vi "StageMoveDone.vi"(8 "error in (no error)":errorcluster, 11 "InterferometryUI in":refnum<class "InterferometryUI.lvclass">) -> (0 "error out":errorcluster, 3 "InterferometryUI out":refnum<class "InterferometryUI.lvclass">)   [LabVIEW 2023, in "InterferometryUI.lvlib" / "InterferometryUI.lvclass"]
uses:
  InterferometryUI.lvclass
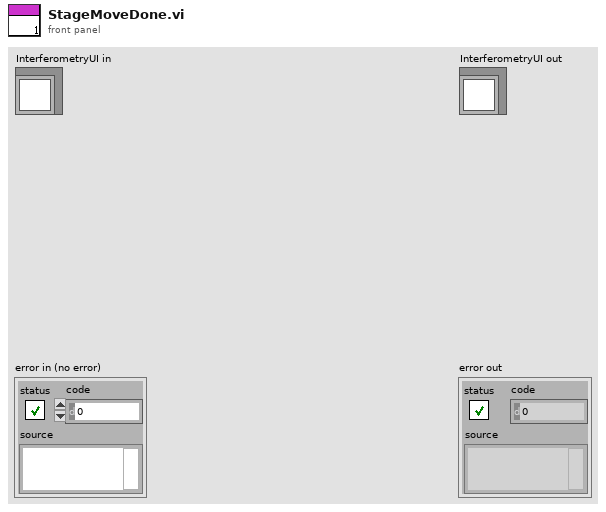
[diagram p1: front panel]
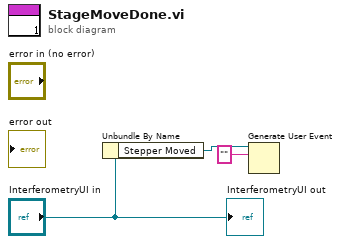
[diagram p0: block diagram]
diagram:
  n1 = Unbundle By Name("InterferometryUI in") -> ("Stepper Moved"=w2:refnum<user-event>)
  n2 = Generate User Event(user event=w2, event data cluster="" ("event data")) -> ()  [unwired: 2 in, 2 out]
  "InterferometryUI out" <- "InterferometryUI in"
